vi "calculoVelocidad.vi"(6 "Resolucion":i32, 7 "primera_iteracion?":bool, 9 "motor_gripper?":bool, 10 "Pasos_anteriores":i32, 11 "Pasos_nuevos":i32) -> (2 "RPM":dbl)   [LabVIEW 2026]
uses:
  GlobalVariable/Muestreo.vi
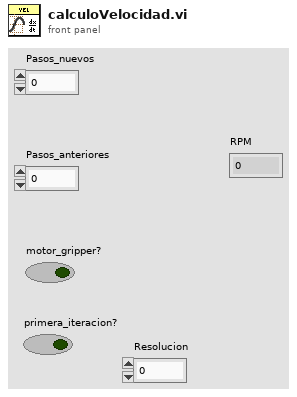
[diagram p1: front panel]
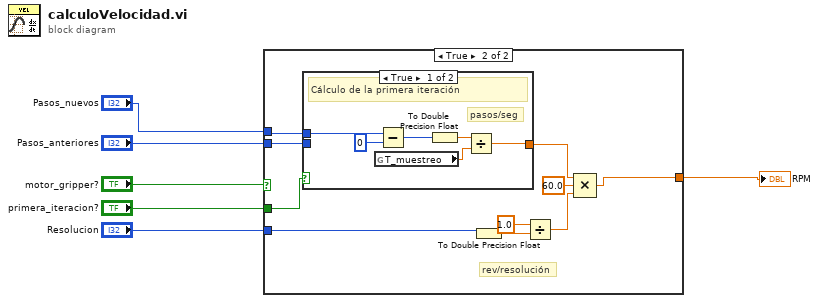
[diagram p0: block diagram]
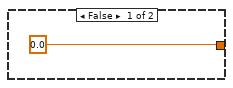
[diagram p2: hidden frame]
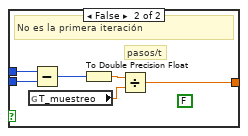
[diagram p3: hidden frame]
diagram:
  n1 = case shown="True" "motor_gripper?" {
    tunnel: "Pasos_anteriores" -> [_ w17]
    tunnel: "Pasos_nuevos" -> [_ w16]
    tunnel: "Resolucion" -> [_ w11]
    tunnel: [0.0 ("mean") w9] -> w5
    tunnel: "primera_iteracion?" -> [_ w8]
    frame False {
    }
    frame True {
      # "rev/resolución"
      n2 = case shown="True" w8 {
        tunnel: w17 -> [_ w29]
        tunnel: w16 -> [w19 w26]
        tunnel: [w20 w24] -> w10
        frame True {
          # "pasos/seg"
          # "Cálculo de la primera iteración"
          n3 = global read "Muestreo.vi" "T_muestreo"() -> (w23:dbl)
          n4 = Subtract(x=w19, y=0) -> (x-y=w21:i32)
          n5 = To Double Precision Float(number=w21) -> (double precision float=w22:dbl)
          n6 = Divide(x=w22, y=w23) -> (x/y=w20:dbl)
        }
        frame False {
          (unwired) FALSE
          # "pasos/t"
          # "No es la primera iteración"
          n7 = global read "Muestreo.vi" "T_muestreo"() -> (w25:dbl)
          n8 = Subtract(x=w26, y=w29) -> (x-y=w28:i32)
          n9 = To Double Precision Float(number=w28) -> (double precision float=w27:dbl)
          n10 = Divide(x=w27, y=w25) -> (x/y=w24:dbl)
        }
      }
      n11 = To Double Precision Float(number=w11) -> (double precision float=w14:dbl)
      n12 = Divide(x=1.0, y=w14) -> (x/y=w15:dbl)
      n13 = Compound Arithmetic op=MULTIPLY(w10, 60.0 ("value"), w15) -> (w9:dbl)
    }
  }
  "RPM" <- w5
